vi "Convert Variant To U16.vi"(10 "error in (no error)":errorcluster, 11 "Variant":variant) -> (2 "error out":errorcluster, 3 "Numeric":u16)   [LabVIEW 2020]
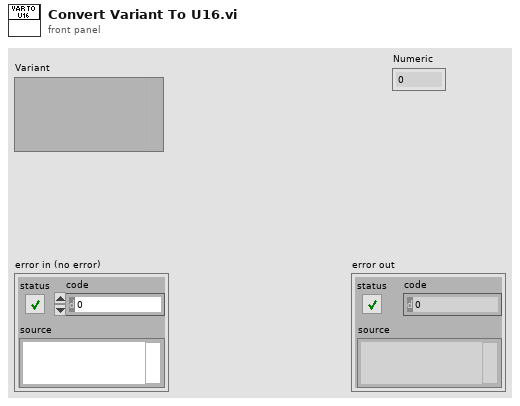
[diagram p1: front panel]
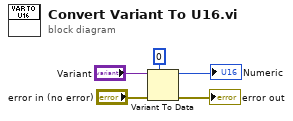
[diagram p0: block diagram]
diagram:
  n1 = Variant To Data(error in="error in (no error)", type=u16 0, Variant="Variant") -> (data=→"Numeric":u16, error out=→"error out":errorcluster)
